vi "Generate Terms XML.vi"(4 "error in (no error)":errorcluster, 6 "Terminals":T1[](array[typedef]), 7 "Node Name":string) -> (0 "error out":errorcluster, 3 "XML out":string)   [LabVIEW 2020, in "Web Service Description.lvlib"]
uses:
  <vilib>/AppBuilder/Engine/WebServiceDescription/Web Service Description.lvlib
  <vilib>/AppBuilder/Engine/WebServiceDescription/Terminal Info.ctl
  <vilib>/AppBuilder/Engine/WebServiceDescription/LVDataTypes/LVType/LVType.lvclass
  <vilib>/AppBuilder/Engine/WebServiceDescription/NextGenXMLTypeGenerator/NextGenXMLTypeGenerator.lvclass
  e:/builds/penguin/labview/branches/2020/dev/dist/vi.lib/AppBuilder/Engine/WebServiceDescription/LVDataTypes/LVTypeVisitor/LVTypeVisitor.lvclass
  <vilib>/AppBuilder/Engine/WebServiceDescription/XMLGen/XMLGen.lvlib
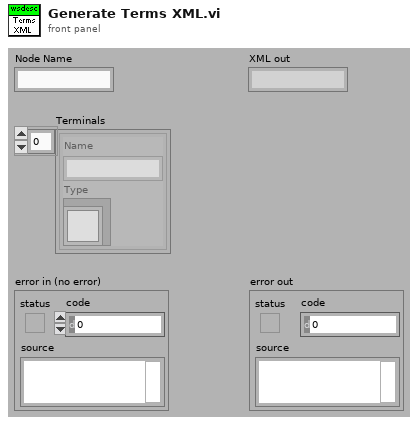
[diagram p1: front panel]
types:
  T1 = typedef "Web Service Description.lvlib/Terminal Info.ctl" = cluster{"Name":string, "Type":refnum<class "LVType.lvclass">}
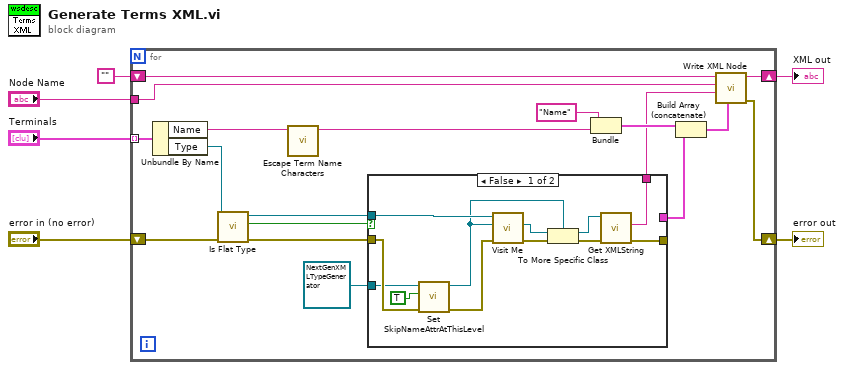
[diagram p0: block diagram]
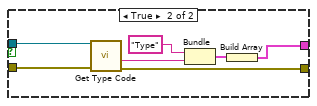
[diagram p2: hidden frame]
diagram:
  n1 = for {
    tunnel: "Terminals" -> [w24] mode=indexing
    shift-right: [w18] -> w5
    shift-left: "" -> [w19]
    shift-right: [w15] -> w4
    shift-left: "error in (no error)" -> [w22]
    tunnel: "Node Name" -> [w9]
    n2 = Unbundle By Name(w24) -> ("Name"=w8:string, "Type"=w23:refnum<class "LVType.lvclass">)
    n3 = call-dynamic "Is Flat Type.vi"("error in (no error)"=w22, "LVType in"=w23) -> ("error out"=w17:errorcluster, "Flat Type?"=w21:bool, "LVType out"=w16:refnum<class "LVType.lvclass">)  [unwired: 7 out]
    n4 = call <vilib>:"Escape Term Name Characters.vi"("terminal name in"=w8) -> ("terminal name out"=w7:string)  [unwired: 10 in]
    n5 = case shown="False" w21 {
      tunnel: w17 -> [w29 w41]
      tunnel: w16 -> [w36 w42]
      tunnel: [_ w38] -> w13
      tunnel: refnum<class "NextGenXMLTypeGenerator.lvclass"> refnum ("NextGenXMLTypeGenerator in") -> [w28 _]
      tunnel: [w31 w37] -> _
      tunnel: [w30 _] -> w10
      frame False {
        n6 = call <vilib>:"Set SkipNameAttrAtThisLevel.vi"("error in (no error)"=w29, "SkipNameAttrAtThisLevel"=TRUE, "NextGenXMLTypeGenerator.lvclass in"=w28) -> ("error out"=w27:errorcluster, "NextGenXMLTypeGenerator.lvclass out"=w26:refnum<class "NextGenXMLTypeGenerator.lvclass">)  [unwired: 7 out]
        n7 = call-dynamic "Visit Me.vi"("error in (no error)"=w27, "Visitor In"=w26, "LVType in"=w36) -> ("error out"=w35:errorcluster, "Visitor Out"=w34:refnum<class "LVTypeVisitor.lvclass">)  [unwired: 7 out]
        n8 = To More Specific Class(target class=w26, reference=w34, error in=w35) -> (specific class reference=w33:refnum<class "NextGenXMLTypeGenerator.lvclass">, error out=w32:errorcluster)
        n9 = call <vilib>:"Get XMLString.vi"("error in (no error)"=w32, "NextGenXMLTypeGenerator.lvclass in"=w33) -> ("error out"=w31:errorcluster, "XMLString"=w30:string)  [unwired: 8 out]
      }
      frame True {
        n10 = call <vilib>:"Get Type Code.vi"("error in (no error)"=w41, "LVType.lvclass in"=w42) -> ("error out"=w37:errorcluster, "TypeCodeString"=w40:string)  [unwired: 8 out]
        n11 = Bundle("Type", "TypeCodeString"=w40) -> (w39:cluster{string, "TypeCodeString":string})  [unwired: 1 out]
        n12 = Build Array(w39) -> (w38:cluster{string, "TypeCodeString":string}[])
      }
    }
    n13 = Bundle("Name", "terminal name out"=w7) -> (w14:cluster{string, "terminal name out":string})  [unwired: 1 out]
    n14 = Build Array (concatenate)(w14, w13) -> (w12:cluster{string, "TypeCodeString":string}[])
    n15 = call <vilib>:"Write XML Node.vi"("attributes"=w12, "body"=w10, "node"=w9, "initial string"=w19) -> ("error out"=w15:errorcluster, "resulting string"=w18:string)  [unwired: 1 in, 5 out]
  }
  "XML out" <- w5
  "error out" <- w4
